vi "FlattenInvaders.vi"(6 "MainCluster _OUT":T9, 11 "Picture_IN":picture) -> (3 "Picture_OUT":picture)   [LabVIEW 2019]
uses:
  InitCluster.ctl
  CharacterCluster.ctl
  <vilib>/picture/picture.llb/imagedata.ctl
  ShotInitCluster.ctl
  <vilib>/Utility/miscctls.llb/LVPositionTypeDef.ctl
  <vilib>/Utility/miscctls.llb/LVBoundsTypeDef.ctl
  InvaderPositionArray.ctl
  move_dir_lr.ctl
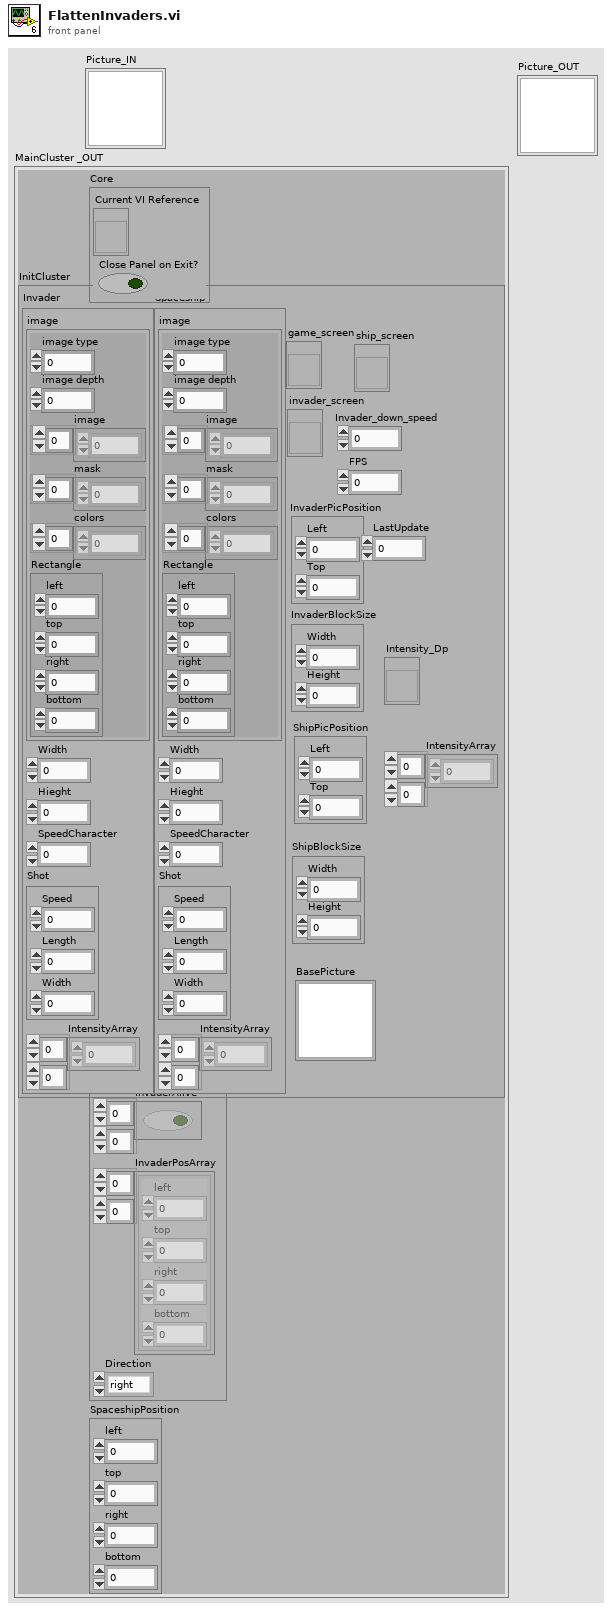
[diagram p1: front panel]
types:
  T1 = typedef "InitCluster.ctl" = cluster{"Invader":T2, "Spaceship":T2, "game_screen":refnum<vi>, "BasePicture":picture, "invader_screen":refnum<vi>, "InvaderPicPosition":T5, "Invader_down_speed":i16, "FPS":u16, "InvaderBlockSize":T6, "ship_screen":refnum<vi>, "ShipBlockSize":T6, "ShipPicPosition":T5, "LastUpdate":u32, "Intensity_Dp":refnum<vi>, "IntensityArray":u8[][]}
  T2 = typedef "CharacterCluster.ctl" = cluster{"image":T3, "Width":u32, "Hieght":u32, "SpeedCharacter":u32, "Shot":T4, "IntensityArray":u8[][]}
  T3 = typedef "imagedata.ctl" = cluster{"image type":i32, "image depth":i32, "image":u8[], "mask":u8[], "colors":u32[], "Rectangle":cluster{"left":i16, "top":i16, "right":i16, "bottom":i16}}
  T4 = typedef "ShotInitCluster.ctl" = cluster{"Speed":u32, "Length":u32, "Width":u32}
  T5 = typedef "LVPositionTypeDef.ctl" = cluster{"Left":i32, "Top":i32}
  T6 = typedef "LVBoundsTypeDef.ctl" = cluster{"Width":u32, "Height":u32}
  T7 = typedef "InvaderPositionArray.ctl" = cluster{"InvaderAlive":bool[][], "InvaderPosArray":cluster{"left":i16, "top":i16, "right":i16, "bottom":i16}[][], "Direction":T8}
  T8 = typedef "move_dir_lr.ctl" = enum16{"right", "left"}
  T9 = cluster{"Core":cluster{"Current VI Reference":refnum<vi>, "Close Panel on Exit?":bool}, "InitCluster":T1, "InvaderPosArray":T7, "SpaceshipPosition":cluster{"left":i16, "top":i16, "right":i16, "bottom":i16}}
  T10 = cluster{"left":i16, "top":i16, "right":i16, "bottom":i16}[][]
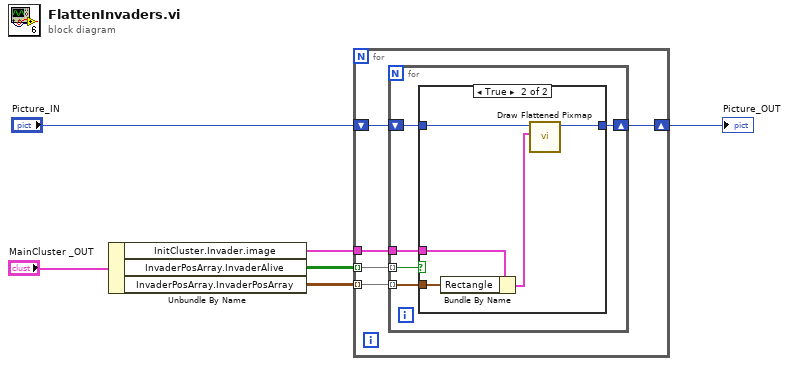
[diagram p0: block diagram]
diagram:
  n1 = Unbundle By Name("MainCluster _OUT") -> ("InitCluster.Invader.image"=w3:T3, "InvaderPosArray.InvaderAlive"=w2:bool[][], "InvaderPosArray.InvaderPosArray"=w1:T10)
  n2 = for {
    shift-right: [w10] -> w5
    shift-left: "Picture_IN" -> [w11]
    tunnel: w3 -> [w9]
    tunnel: w2 -> [w8] mode=indexing
    tunnel: w1 -> [w7] mode=indexing
    n3 = for {
      tunnel: w9 -> [w14]
      tunnel: w8 -> [w13] mode=indexing
      shift-right: [w15] -> w10
      shift-left: w11 -> [w16]
      tunnel: w7 -> [w12] mode=indexing
      n4 = case shown="True" w13 {
        tunnel: w16 -> [w17 w22]
        tunnel: [w17 w21] -> w15
        tunnel: w14 -> [_ w20]
        tunnel: w12 -> [_ w18]
        frame False {
        }
        frame True {
          n5 = Bundle By Name(cluster=w20, "Rectangle"=w18) -> (w19:T3)
          n6 = call <vilib>:"Draw Flattened Pixmap.vi"("image data"=w19, "picture"=w22) -> ("new picture"=w21:picture)  [unwired: 7 in]
        }
      }
    }
  }
  "Picture_OUT" <- w5
